vi "ParseFIFO_HH.vi"(2 "RawData":u32[](array[numeric])) -> (0 "RawData Out":T1)   [LabVIEW 2009]
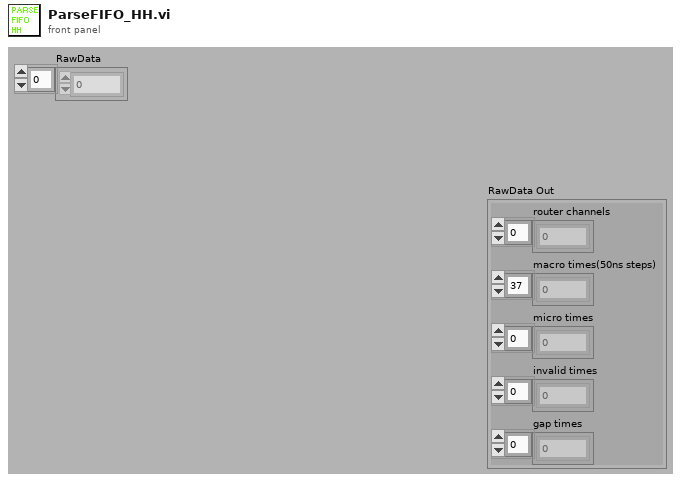
[diagram p1: front panel]
types:
  T1 = cluster{"router channels":u8[], "macro times(50ns steps)":u32[], "micro times":u16[], "invalid times":u32[], "gap times":u32[]}
  T2 = cluster{"router channels":u8[], "macro times (50ns steps)":u32[], "micro times":u16[], "invalid times":u32[], "gap times":u32[]}
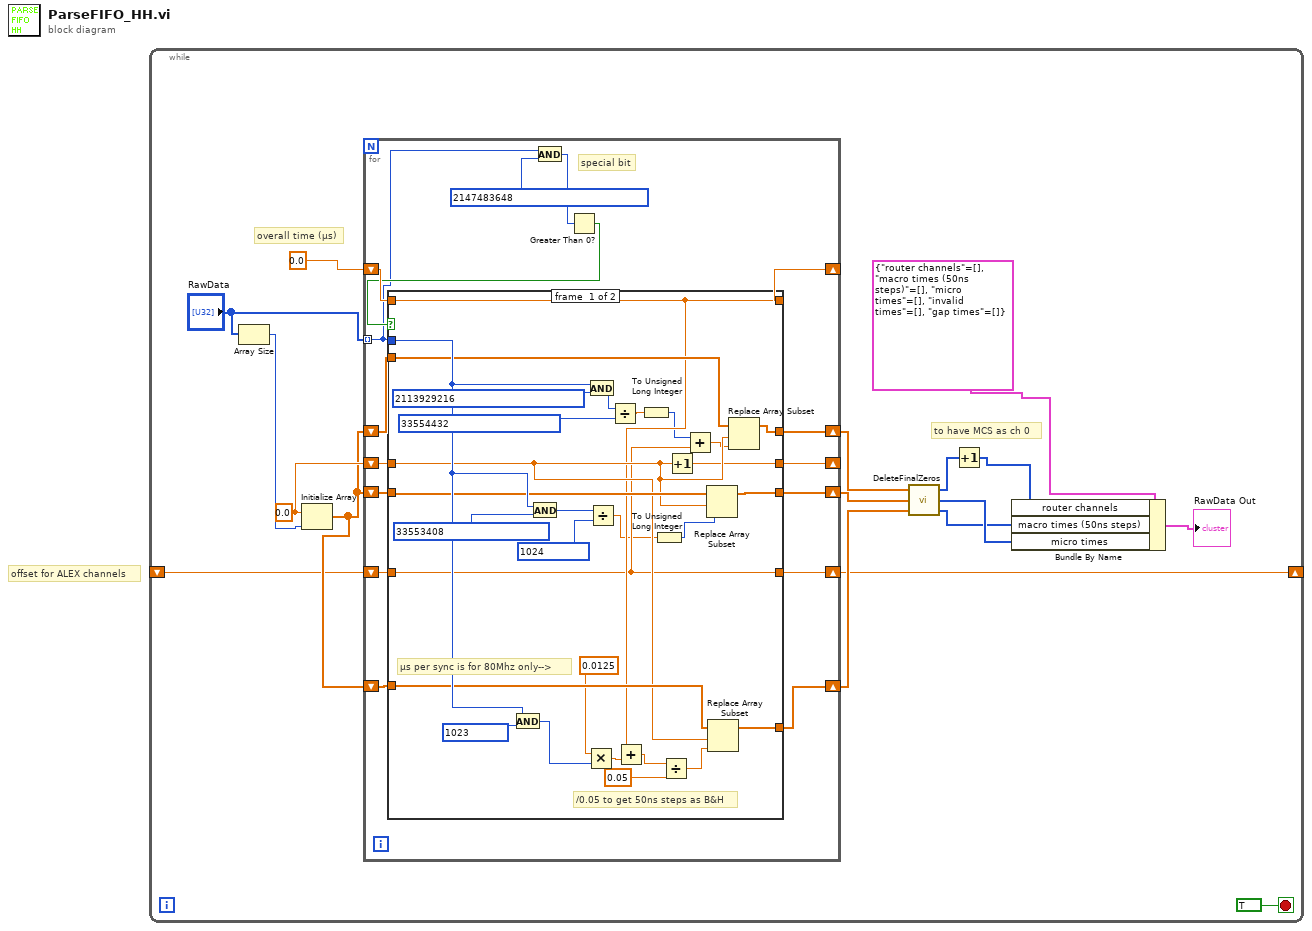
[diagram p0: block diagram]
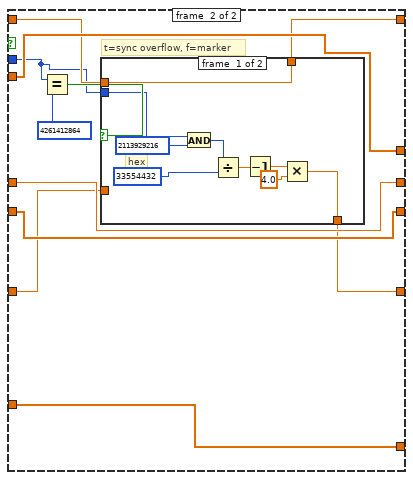
[diagram p2: hidden frame]
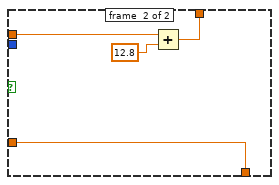
[diagram p3: hidden frame]
diagram:
  # "offset for ALEX channels"
  n1 = while {
    shift-right: [w2] -> _
    shift-left: _ -> [w5]
    stop <- TRUE stop-if-true
    w17 = 0.0 ("Element")
    # "overall time (µs)"
    # "to have MCS as ch 0"
    n2 = Array Size(array="RawData") -> (size(s)=w13:i32)
    n3 = Initialize Array(w17, w13) -> (w6:dbl[])
    n4 = for {
      tunnel: "RawData" -> [w28] mode=indexing
      shift-right: [w32] -> _
      shift-left: 0.0 -> [w33]
      shift-right: [w22] -> w4
      shift-left: w6 -> [w23]
      shift-right: [w24] -> w16
      shift-left: w6 -> [w25]
      shift-right: [w26] -> w15
      shift-left: w6 -> [w27]
      shift-right: [w20] -> _
      shift-left: w17 -> [w21]
      shift-right: [w18] -> w2
      shift-left: w5 -> [w19]
      # "special bit"
      n5 = And(x=w28, y=u32 2147483648) -> (x .and. y?=w30:u32)
      n6 = Greater Than 0?(x=w30) -> (x > 0?=w29:bool)
      n7 = case shown="False" w29 {
        tunnel: w33 -> [w41 w68]
        tunnel: [w41 w69] -> w32
        tunnel: w28 -> [w56 w65]
        tunnel: w27 -> [w55 w73]
        tunnel: [w54 w73] -> w26
        tunnel: w25 -> [w53 w72]
        tunnel: [w52 w72] -> w24
        tunnel: w23 -> [w51 w71]
        tunnel: [w50 w71] -> w22
        tunnel: w21 -> [w49 w70]
        tunnel: [w48 w70] -> w20
        tunnel: w19 -> [w38 w63]
        tunnel: [w38 w64] -> w18
        frame #0 {
          # "/0.05 to get 50ns steps as B&H"
          # "µs per sync is for 80Mhz only-->"
          n8 = And(x=w56, y=u32 1023) -> (x .and. y?=w39:u32)
          n9 = And(x=w56, y=u32 33553408) -> (x .and. y?=w45:u32)
          n10 = Multiply(x=0.0125, y=w39) -> (x*y=w47:dbl)
          n11 = And(x=w56, y=u32 2113929216) -> (x .and. y?=w58:u32)
          n12 = Divide(x=w45, y=u32 1024) -> (x/y=w37:dbl)
          n13 = Divide(x=w58, y=u32 33554432) -> (x/y=w60:dbl)
          n14 = Add(x=w41, y=w47) -> (x+y=w43:dbl)
          n15 = To Unsigned Long Integer(number=w60) -> (unsigned 32bit integer=w35:u32)
          n16 = To Unsigned Long Integer(number=w37) -> (unsigned 32bit integer=w36:u32)
          n17 = Divide(x=w43, y=0.05) -> (x/y=w40:dbl)
          n18 = Increment(x=w49) -> (x+1=w48:dbl)
          n19 = Add(x=w35, y=w38) -> (x+y=w34:dbl)
          n20 = Replace Array Subset(array=w53, new element=w36, index=w49) -> (w52:dbl[])
          n21 = Replace Array Subset(array=w51, new element=w40, index=w49) -> (w50:dbl[])
          n22 = Replace Array Subset(array=w55, new element=w34, index=w49) -> (w54:dbl[])
        }
        frame #1 {
          # "t=sync overflow, f=marker"
          n23 = Equal?(x=w65, y=u32 4261412864) -> (x = y?=w66:bool)
          n24 = case shown="True" w66 {
            tunnel: [w78 w85] -> w69
            tunnel: w68 -> [w78 w84]
            tunnel: w65 -> [w82 _]
            tunnel: [w74 w83] -> w64
            tunnel: w63 -> [_ w83]
            frame #0 {
              # "hex"
              n25 = And(x=w82, y=u32 2113929216) -> (x .and. y?=w80:u32)
              n26 = Divide(x=w80, y=u32 33554432) -> (x/y=w77:dbl)
              n27 = Decrement(x=w77) -> (x-1=w76:dbl)
              n28 = Multiply(x=w76, y=4.0) -> (x*y=w74:dbl)
            }
            frame #1 {
              n29 = Add(x=w84, y=12.8) -> (x+y=w85:dbl)
            }
          }
        }
      }
    }
    n30 = call "DeleteFinalZeros.vi"("in MacroTime"=w4, "in MicroTime"=w16, "in channel"=w15) -> ("out MacroTime"=w3:u32[], "out MicroTime"=w8:u32[], "out channel"=w9:u32[])
    n31 = Increment(x=w9) -> (x+1=w7:u32[])
    n32 = Bundle By Name(cluster=T2 {"router channels"=[], "macro times (50ns steps)"=[], "micro times"=[], "invalid times"=[], "gap times"=[]} ("rawdata"), "router channels"=w7, "macro times (50ns steps)"=w3, "micro times"=w8) -> (→"RawData Out":T2)
  }
